vi "Dismiss Error.vi"(8 "error in (no error)":errorcluster, 10 "Select Error":i32, 11 "Error Manager in":refnum<class "Error Manager.lvclass">) -> (0 "error out":errorcluster, 3 "Error Manager out":refnum<class "Error Manager.lvclass">)   [LabVIEW 2026, in "TALOS.lvlib" / "Error Manager.lvlib" / "Error Manager.lvclass"]
uses:
  Error Manager.lvclass
  C:/LabVIEW Code/TALOS/talos/Father of all uServices/Father of all uServices/Father of all uServices.lvclass
  Error Manager.lvclass/Error Manager.ctl
  Father of all uServices/Father of all uServices/Father of all uServices.lvclass/Father of all uServices.ctl
  Ancestor/Ancestor/Ancestor.lvclass/Ancestor.ctl
  Common GUI v3/Common GUI v3/Error Listbox Msg.ctl
  Common GUI v3/Common GUI v3/Error Listbox Msg Action.ctl
  Error Info.ctl
  Guardian/Guardian/Requests.ctl
  Guardian/Guardian Messages/Requests from uServices Msg/Requests from uServices Msg.lvclass/Requests from uServices Msg.ctl
  Guardian/Guardian Messages/Requests from uServices Msg/Send Requests from uServices.vi
  Support VIs/Generate Error.vi
  FGV/Error Memory/Get Error Description.vi
  Support VIs/Get PC name.vi
  Ancestor/Ancestor/Read ID.vi
  Support VIs/Get Class Name.vi
  <vilib>/Utility/error.llb/Clear Errors.vi
  FGV/Error Memory/Error Memory Core.vi
  <vilib>/AdvancedString/Delimited String to 1D String Array.vi
  <vilib>/AdvancedString/Delimited String to 1D String Array (string).vi
  Support VIs/Circus Root Path.vi
  FGV/Error Memory/Error Crt Lvl checker.vi
  FGV/Error Memory/Error Memory Core.vi/40c8088d-b597-4017-91af-faa98e00292e.vi
  FGV/Error Memory/Error Memory Core.vi/d4a3ab98-063c-4e44-b43d-fbdcfe6c2be2.vi
  Father of all uServices/Father of all uServices/Father of all uServices.lvclass
  C:/LabVIEW Code/TALOS/builds/Actor Framework PPL/Actor Framework.lvlibp/1abvi3w/vi.lib/ActorFramework/Actor/Actor.lvclass
  Support VIs/Global Memory.vi
  <vilib>/Utility/LVClass/Get LV Class Name.vi
  Support VIs/Is in Packed Library.vi
  Support VIs/TALOS Root path.vi
  Support VIs/Read CSV worksheet.vi
  Support VIs/Global Constants.vi
  <vilib>/Utility/error.llb/General Error Handler.vi
  Support VIs/Error Log.vi
  builds/Actor Framework PPL/Actor Framework.lvlibp/1abvi3w/vi.lib/ActorFramework/Actor/Read Caller Enqueuer.vi
  builds/Actor Framework PPL/Actor Framework.lvlibp/1abvi3w/vi.lib/ActorFramework/Message Enqueuer/Enqueue.vi
  Ancestor/Ancestor/Ancestor.lvclass
  <vilib>/Comparison/Equal/Equal Functor/Equal Functor.lvclass
  Guardian/Guardian Messages/Requests from uServices Msg/Requests from uServices Msg.lvclass
  Guardian/Guardian/Guardian.lvclass
  Common GUI v3/Common GUI v3/Common GUI v3.lvclass
  TALOS.lvlib
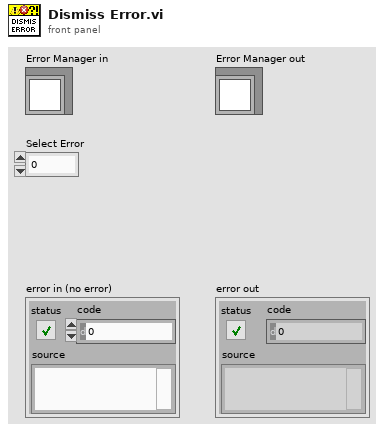
[diagram p1: front panel]
types:
  T1 = typedef "TALOS.lvlib/Guardian.lvlib/Guardian.lvclass/Requests.ctl" = enum16{"Ready to Launch", "Start RUN", "Stop RUN", "Update DAQ Params", "Update Error Listbox", "Update Run Status", "Update Kasli Log", "Run Stopped with Errors", "Switch uS View", "Dismiss All Errors"}
  T2 = typedef "TALOS.lvlib/Common GUI v3.lvlib/Common GUI v3.lvclass/Error Listbox Msg Action.ctl" = enum16{"Add", "Remove", "Clear"}
  T3 = typedef "TALOS.lvlib/Common GUI v3.lvlib/Common GUI v3.lvclass/Error Listbox Msg.ctl" = cluster{"Action":T2, "Error Info":T4}
  T4 = typedef "TALOS.lvlib/Error Manager.lvlib/Error Manager.lvclass/Error Info.ctl" = cluster{"error out":errorcluster, "Time Stamp":timestamp, "Machine Name":string, "GUID":string}
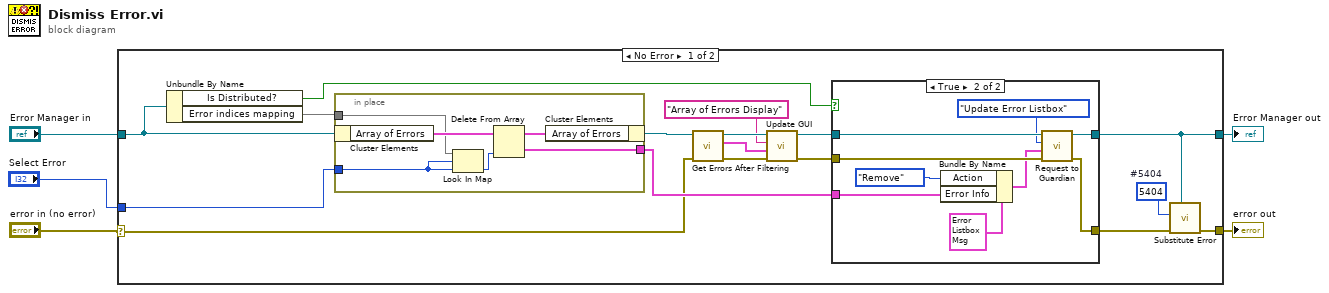
[diagram p0: block diagram]
diagram:
  n1 = case shown="No Error" "error in (no error)" {
    selector: "error in (no error)" -> [w12 w40]
    tunnel: "Error Manager in" -> [w20 w41]
    tunnel: [w7 w40] -> w1
    tunnel: [w6 w41] -> w4
    tunnel: "Select Error" -> [w11 _]
    frame No Error {
      w9 = 5404  # #5404
      n2 = Unbundle By Name(w20) -> ("Is Distributed?"=w10:bool, "Error indices mapping"=w21:map{i32, i32})
      n3 = in-place {
        in-place-border: w21 -> [w36]
        in-place-border: [w35] -> w22
        in-place-border: w11 -> [w34]
        n4 = in-place-cluster #1(w20) -> ("Array of Errors"=w39:T4[])
        n5 = Look In Map(map=w36, key=w34, default value=w34) -> (value=w37:i32)  [unwired: 1 out]
        n6 = Delete From Array(array=w39, index=w37) -> (deleted portion=w35:T4, array with subset deleted=w38:T4[])  [unwired: 1 in]
        n7 = in-place-cluster #1("Array of Errors"=w38) -> (w14:refnum<class "Error Manager.lvclass">)
      }
      n8 = call-dynamic "Get Errors After Filtering.vi"("error in (no error)"=w12, "Error Manager in"=w14) -> ("error out"=w17:errorcluster, "Array of Errors"=w16:T4[], "Error Manager out"=w15:refnum<class "Error Manager.lvclass">)  [unwired: 7 in]
      n9 = call "Update GUI.vi"("error in (no error)"=w17, "Data"=w16, "GUI Item Name"="Array of Errors Display" ("FP Item Name"), "uService Template in"=w15) -> ("error out"=w19:errorcluster, "uService Template out"=w18:refnum<class "Error Manager.lvclass">)  [unwired: 6 in]
      n10 = case shown="True" w10 {
        tunnel: w22 -> [_ w33]
        tunnel: w19 -> [w23 w32]
        tunnel: w18 -> [w24 w31]
        tunnel: [w23 w30] -> w8
        tunnel: [w24 w26] -> w6
        frame False {
        }
        frame True {
          n11 = Bundle By Name(cluster=T3 {"Action"=enum."Add", "Error Info"={"error out"={"status"=FALSE, "code"=0, "source"=""}, "Time Stamp"=timestamp(0 s since 1904-01-01), "Machine Name"="", "GUID"=""}} ("Error Listbox Msg"), "Action"=Error_Listbox_Msg_Action."Remove", "Error Info"=w33) -> (w29:T3)
          n12 = call "Request to Guardian.vi"("error in (no error)"=w32, "Data"=w29, "Requests"=Requests."Update Error Listbox", "Father of all uServices in"=w31) -> ("error out"=w30:errorcluster, "Father of all uServices out"=w26:refnum<class "Error Manager.lvclass">)  [unwired: 6 in]
        }
      }
      n13 = call "Substitute Error.vi"("LabVIEW Object"=w6, "error in (no error)"=w8, "Error Code"=w9) -> ("error out"=w7:errorcluster)  [unwired: 8 in]
    }
    frame Error {
    }
  }
  "error out" <- w1
  "Error Manager out" <- w4
